vi "prompt_user_for_projector_settings.vi"() -> (0 "blue exp_time_us out":i32=8215, 1 "red exp_time_us out":i32=8215, 2 "green exp_time_us out":i32=235, 3 "RedCurrent out":u8=104, 4 "RedBluePatternRepeat out":i32, 5 "GreenCurrent out":u8=135, 7 "BlueCurrent out":u8=130, 11 "projector params to save":string[][](array[string]))   [LabVIEW 2019]
uses:
  ParametersGlobal.vi
panel:
  in  "RedBluePatternRepeat":i32=2
  in  "OK Button":bool
  in  "BlueCurrent":u8=255
  in  "GreenCurrent":u8=255
  in  "RedCurrent":u8=255
  in  "blue exp_time_us":i32=8274
  in  "red exp_time_us":i32=8274
  in  "green exp_time_us":i32=239
  # "Enter Projector\nSettings for\nThis Computer"
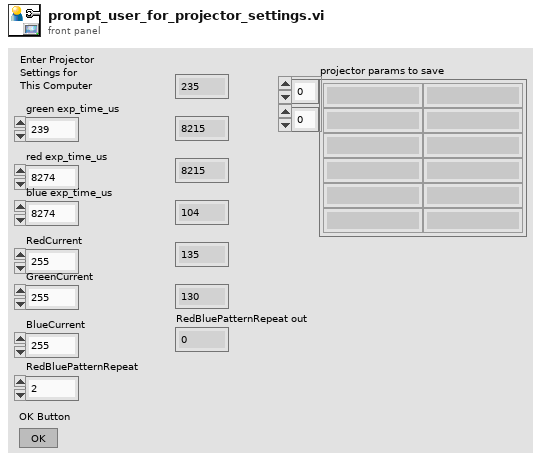
[diagram p1: front panel]
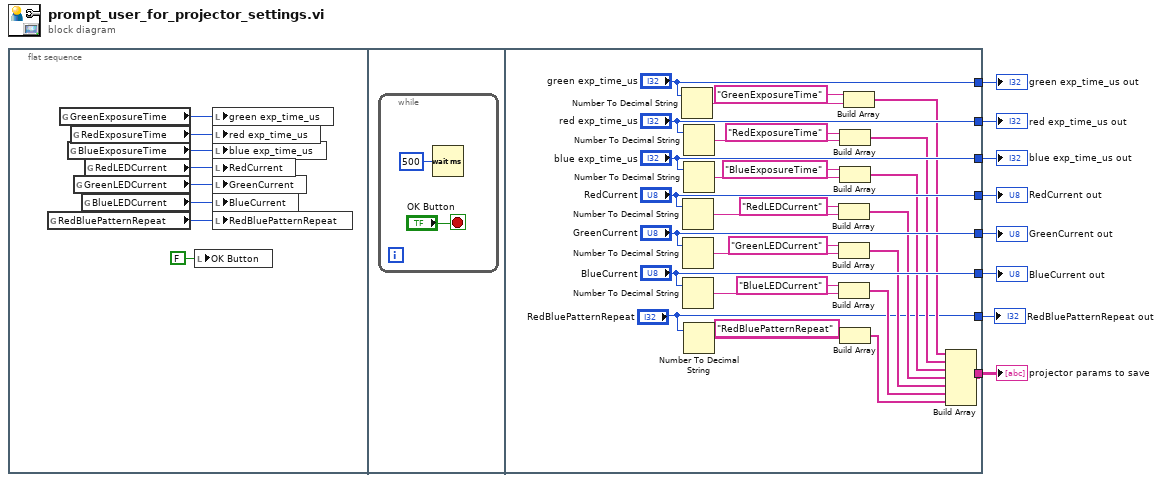
[diagram p0: block diagram]
diagram:
  n1 = flat-sequence {
    tunnel: ["green exp_time_us"] -> w8
    tunnel: ["red exp_time_us"] -> w7
    tunnel: ["blue exp_time_us"] -> w6
    tunnel: ["RedCurrent"] -> w5
    tunnel: ["GreenCurrent"] -> w4
    tunnel: ["BlueCurrent"] -> w3
    tunnel: [w25] -> w2
    tunnel: ["RedBluePatternRepeat"] -> w1
    frame #0 {
      n2 = global read "ParametersGlobal.vi" "RedBluePatternRepeat"() -> (w9:i32)
      n3 = global read "ParametersGlobal.vi" "GreenExposureTime"() -> (w15:i32)
      n4 = global read "ParametersGlobal.vi" "BlueExposureTime"() -> (w13:i32)
      n5 = global read "ParametersGlobal.vi" "RedExposureTime"() -> (w14:i32)
      n6 = global read "ParametersGlobal.vi" "GreenLEDCurrent"() -> (w11:u8)
      n7 = global read "ParametersGlobal.vi" "BlueLEDCurrent"() -> (w10:u8)
      n8 = global read "ParametersGlobal.vi" "RedLEDCurrent"() -> (w12:u8)
      n9 = local write "OK Button"(FALSE ("OK Button")) -> ()
      n10 = local write "green exp_time_us"(w15) -> ()
      n11 = local write "red exp_time_us"(w14) -> ()
      n12 = local write "blue exp_time_us"(w13) -> ()
      n13 = local write "RedCurrent"(w12) -> ()
      n14 = local write "GreenCurrent"(w11) -> ()
      n15 = local write "BlueCurrent"(w10) -> ()
      n16 = local write "RedBluePatternRepeat"(w9) -> ()
    }
    frame #1 {
      n17 = while {
        stop <- "OK Button" stop-if-true
        n18 = Wait (ms)(milliseconds to wait=u32 500) -> ()  [unwired: 1 out]
      }
    }
    frame #2 {
      n19 = Number To Decimal String(number="green exp_time_us") -> (decimal integer string=w45:string)  [unwired: 1 in]
      n20 = Number To Decimal String(number="RedCurrent") -> (decimal integer string=w38:string)  [unwired: 1 in]
      n21 = Number To Decimal String(number="GreenCurrent") -> (decimal integer string=w35:string)  [unwired: 1 in]
      n22 = Number To Decimal String(number="BlueCurrent") -> (decimal integer string=w32:string)  [unwired: 1 in]
      n23 = Number To Decimal String(number="red exp_time_us") -> (decimal integer string=w42:string)  [unwired: 1 in]
      n24 = Number To Decimal String(number="blue exp_time_us") -> (decimal integer string=w41:string)  [unwired: 1 in]
      n25 = Number To Decimal String(number="RedBluePatternRepeat") -> (decimal integer string=w22:string)  [unwired: 1 in]
      n26 = Build Array("RedLEDCurrent", w38) -> (w26:string[])
      n27 = Build Array("GreenLEDCurrent", w35) -> (w24:string[])
      n28 = Build Array("BlueLEDCurrent", w32) -> (w23:string[])
      n29 = Build Array("RedExposureTime", w42) -> (w28:string[])
      n30 = Build Array("BlueExposureTime", w41) -> (w27:string[])
      n31 = Build Array("RedBluePatternRepeat", w22) -> (w19:string[])
      n32 = Build Array("GreenExposureTime", w45) -> (w29:string[])
      n33 = Build Array(w29, w28, w27, w26, w24, w23, w19) -> (w25:string[][])
    }
  }
  "green exp_time_us out" <- w8
  "red exp_time_us out" <- w7
  "blue exp_time_us out" <- w6
  "RedCurrent out" <- w5
  "GreenCurrent out" <- w4
  "BlueCurrent out" <- w3
  "projector params to save" <- w2
  "RedBluePatternRepeat out" <- w1
